vi "main.vi"() -> ()   [LabVIEW 2016]
uses:
  SALEvents/SAL_Events.lvclass
  SALListener/SAL_Listener.lvclass
  SALListener/SAL_Listener.lvclass/SAL_Listener.ctl
  SALEvents/SAL_Events.lvclass/SAL_Events.ctl
  SALLV_dome/DataTypes/command_start.ctl
  SALLV_dome/DataTypes/command_enable.ctl
  SALLV_dome/DataTypes/command_disable.ctl
  SALLV_dome/DataTypes/command_exitControl.ctl
  SALLV_dome/DataTypes/command_standby.ctl
  SALLV_dome/DataTypes/command_SetLouvers.ctl
  SALLV_dome/DataTypes/command_Move.ctl
  SALLV_dome/DataTypes/command_Crawl.ctl
  SALLV_dome/SALLV_dome.lvlib
panel:
  out "position_cmd":sgl
  out "position_actual":sgl
  out "position_error":sgl
  in  "Elevation":dbl
  in  "Azimuth":dbl
  in  "Crawl":bool
  in  "Move":bool
  in  "SetLouvers":bool
  in  "Array":i32[][](array[numeric])
  out "StateValue":string
  out "SummaryState":string
  in  "standby":bool
  in  "exitControl":bool
  in  "disable":bool
  in  "enable":bool
  in  "start":bool
  # "Main Controls"
  # "Louvers Command"
  # "States"
  # "Move Command"
  # "ADB Status"
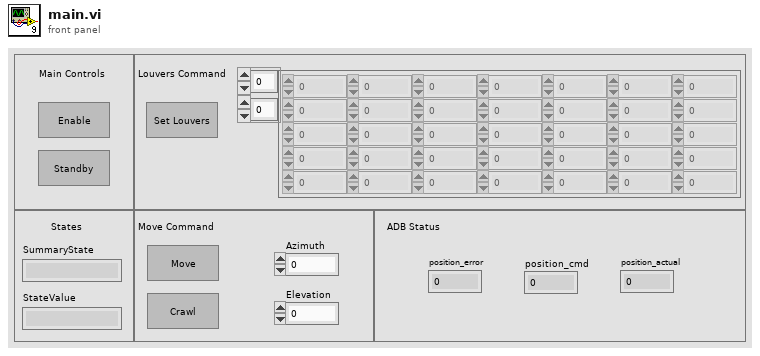
[diagram p1: front panel]
types:
  T1 = typedef "commandsEvents.ctl" = cluster{"start":refnum<user-event>, "disable":refnum<user-event>, "enable":refnum<user-event>, "exitControl":refnum<user-event>, "standby":refnum<user-event>, "stop":refnum<user-event>, "move":refnum<user-event>, "crawl":refnum<user-event>, "setLouvers":refnum<user-event>, "Park":refnum<user-event>, "StopShutter":refnum<user-event>, "OpenShutter":refnum<user-event>, "CloseShutter":refnum<user-event>}
  T2 = typedef "eventsEvents.ctl" = cluster{"AppliedSettingsMatchStart":refnum<user-event>, "ErrorCode":refnum<user-event>, "SettingVersions":refnum<user-event>, "StateChanged":refnum<user-event>, "SummaryState":refnum<user-event>}
  T3 = typedef "telemetryEvents.ctl" = cluster{"ADBstatus":refnum<user-event>}
  T4 = typedef "SALLV_dome.lvlib/command_start.ctl" = cluster{"configuration":string}
  T5 = typedef "SALLV_dome.lvlib/command_enable.ctl" = cluster{"state":bool}
  T6 = typedef "SALLV_dome.lvlib/command_disable.ctl" = cluster{"state":bool}
  T7 = typedef "SALLV_dome.lvlib/command_exitControl.ctl" = cluster{"state":bool}
  T8 = typedef "SALLV_dome.lvlib/command_standby.ctl" = cluster{"state":bool}
  T9 = typedef "SALLV_dome.lvlib/command_SetLouvers.ctl" = cluster{"position[34]":i32[]}
  T10 = typedef "SALLV_dome.lvlib/command_Move.ctl" = cluster{"azimuth":dbl, "elevation":dbl}
  T11 = typedef "SALLV_dome.lvlib/command_Crawl.ctl" = cluster{"azPosition":dbl, "elPosition":dbl, "demandTime":i32}
  T12 = enum16{"", "DisabledState", "EnabledState", "FaultState", "OfflineState", "StandbyState"}
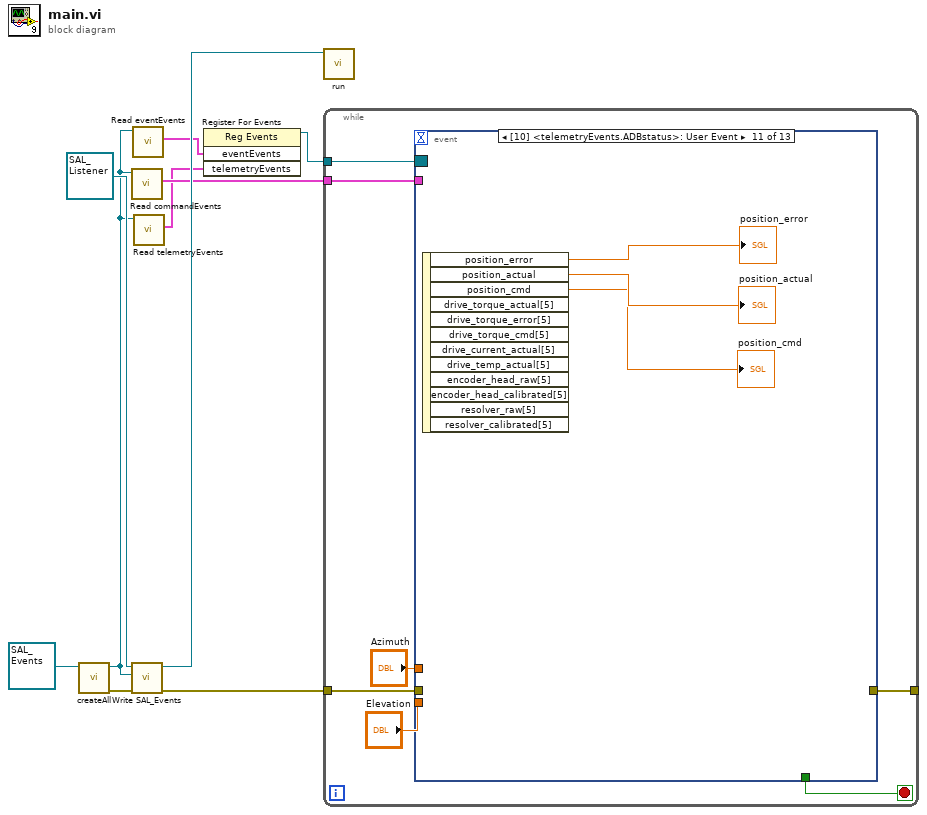
[diagram p0: block diagram]
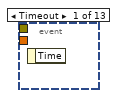
[diagram p2: hidden frame]
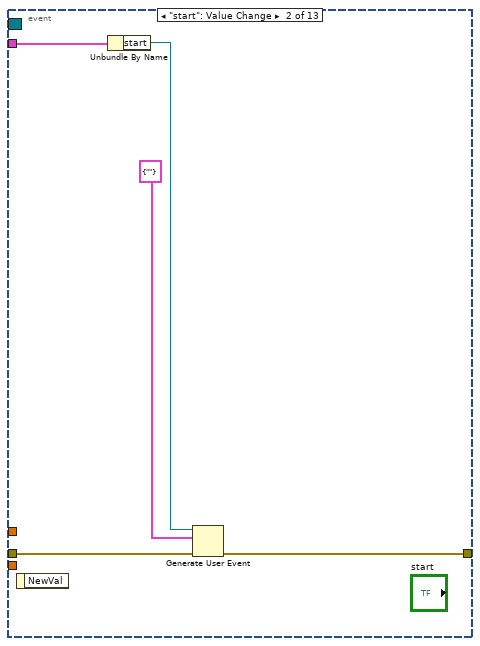
[diagram p3: hidden frame]
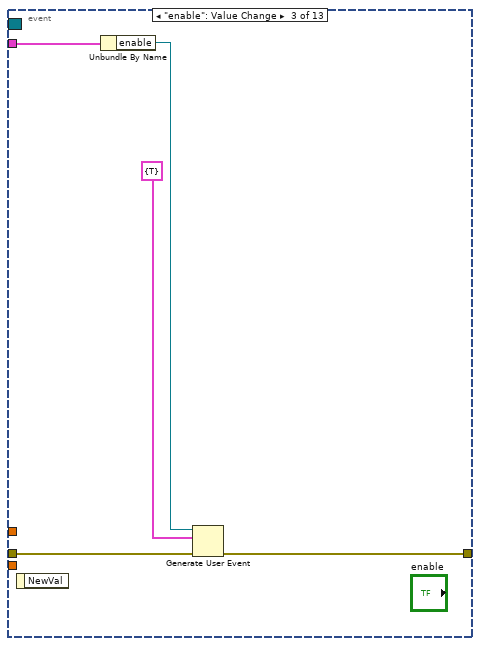
[diagram p4: hidden frame]
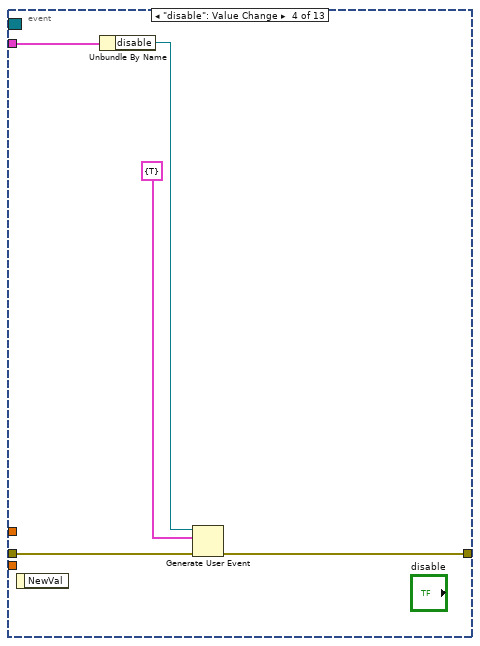
[diagram p5: hidden frame]
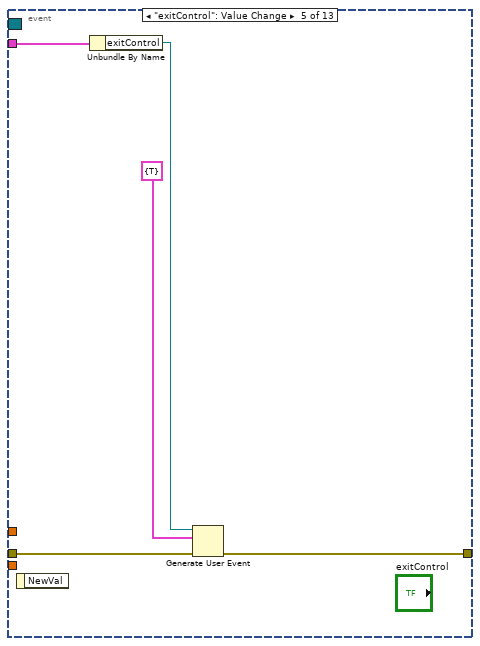
[diagram p6: hidden frame]
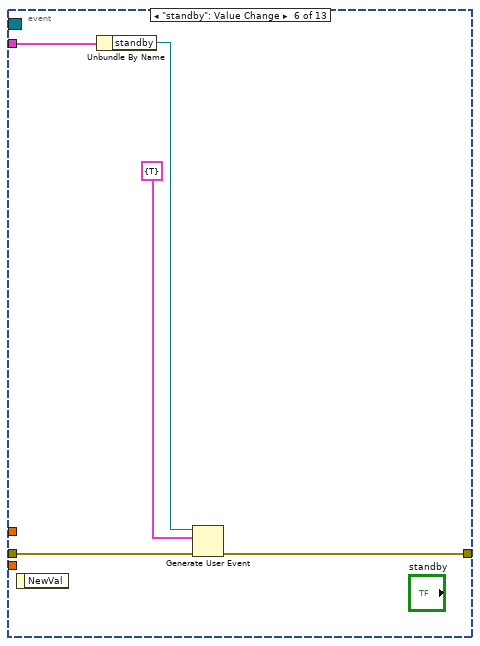
[diagram p7: hidden frame]
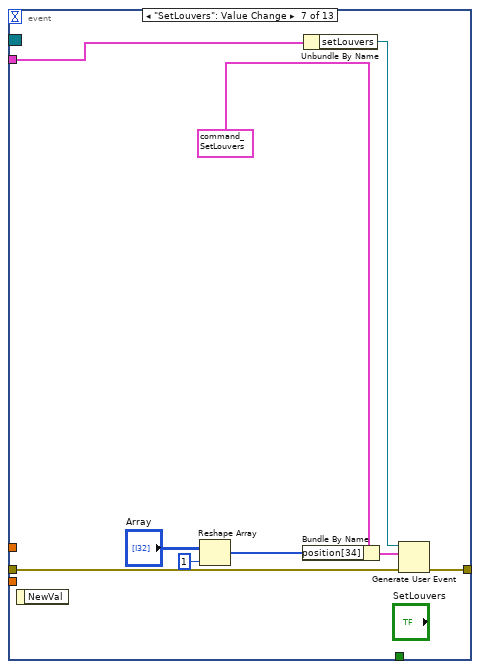
[diagram p8: hidden frame]
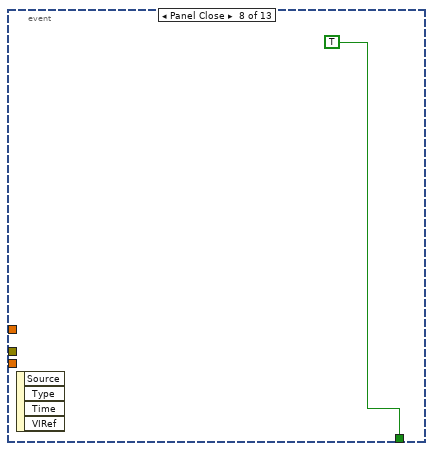
[diagram p9: hidden frame]
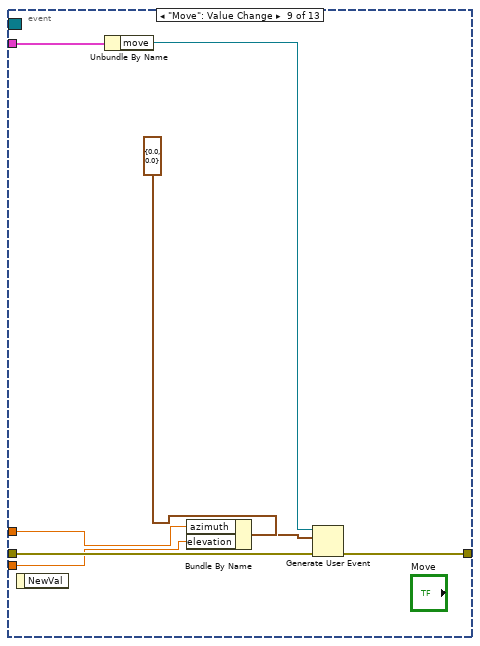
[diagram p10: hidden frame]
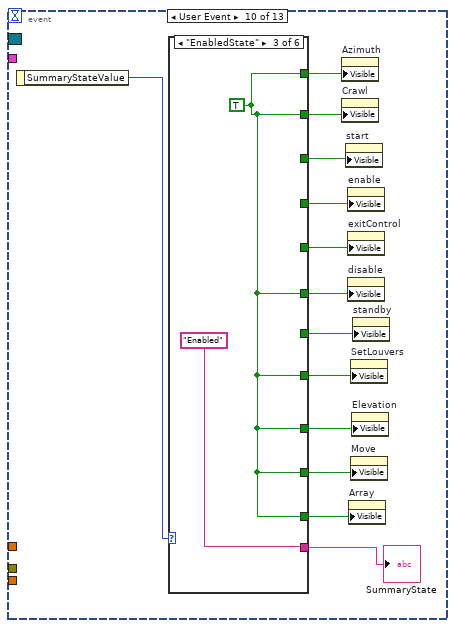
[diagram p11: hidden frame]
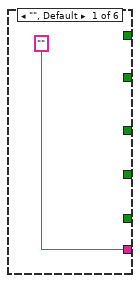
[diagram p12: hidden frame]
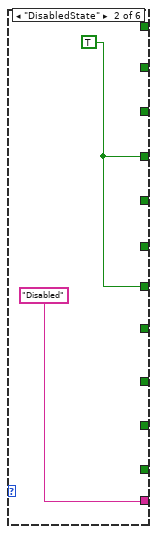
[diagram p13: hidden frame]
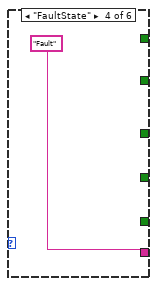
[diagram p14: hidden frame]
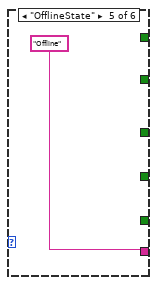
[diagram p15: hidden frame]
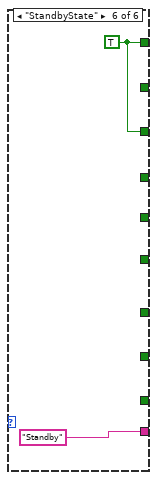
[diagram p16: hidden frame]
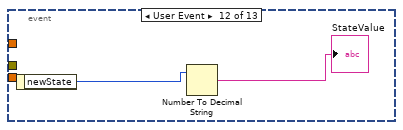
[diagram p17: hidden frame]
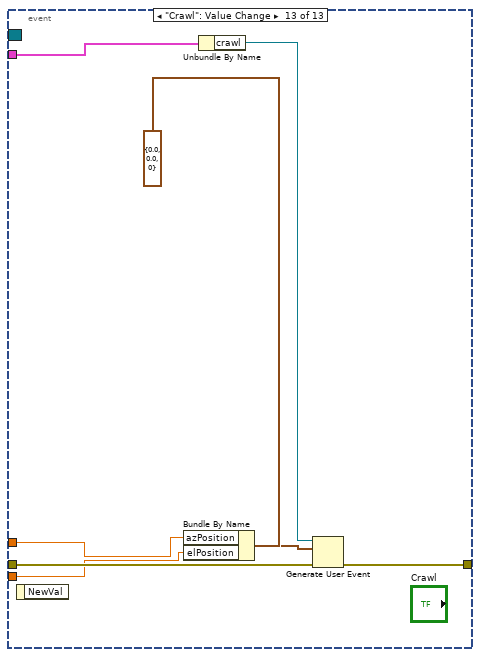
[diagram p18: hidden frame]
diagram:
  n1 = call "createAll.vi"("SAL_Events in"=refnum<class "SAL_Events.lvclass"> refnum ("SAL_Events.lvclass")) -> ("error out"=w7:errorcluster, "SAL_Events out"=w2:refnum<class "SAL_Events.lvclass">)  [unwired: 9 in]
  n2 = call "Read commandEvents.vi"("SAL_Events in"=w2) -> ("commandEvents"=w5:T1)  [unwired: 8 in, 2 out]
  n3 = call "Write SAL_Events.vi"("error in (no error)"=w7, "SAL_Events.lvclass"=w2, "SAL_Listener in"=refnum<class "SAL_Listener.lvclass"> refnum ("SAL_Listener.lvclass")) -> ("error out"=w6:errorcluster, "SAL_Listener out"=w8:refnum<class "SAL_Listener.lvclass">)  [unwired: 7 in]
  n4 = call "Read eventEvents.vi"("SAL_Events in"=w2) -> ("eventEvents"=w4:T2)  [unwired: 8 in, 2 out]
  n5 = call "Read telemetryEvents.vi"("SAL_Events in"=w2) -> ("telemetryEvents"=w1:T3)  [unwired: 8 in, 2 out]
  n6 = register-events(w4, w1) -> (reference out=w3:refnum<event-registration>)  [unwired: 2 in, 1 out]
  n7 = call "run.vi"("SAL_Listener in"=w8) -> ()  [unwired: 9 in, 2 out]
  n8 = while {
    tunnel: w6 -> [w16]
    tunnel: w5 -> [w17]
    tunnel: [w15] -> _
    tunnel: w3 -> [w12]
    stop <- w11 stop-if-true
    n9 = event shown="[10] <telemetryEvents.ADBstatus>: User Event" {
      selector: w12 -> [_ _ _ _ _ _ _ _ _ _ _ _ _]
      dyn-events: _ -> [_ _ _ _ _ _ _ _ _ _ _ _ _]
      timeout: _ -> [_ _ _ _ _ _ _ _ _ _ _ _ _]
      tunnel: w17 -> [_ w22 w27 w32 w37 w42 w51 _ w60 _ _ _ w95]
      tunnel: w16 -> [_ w19 w26 w29 w34 w39 w45 _ w58 _ _ _ w93]
      tunnel: [_ w18 w23 w28 w33 w38 w44 _ w57 _ _ _ w92] -> w15
      tunnel: "Azimuth" -> [_ _ _ _ _ _ _ _ w54 _ _ _ w89]
      tunnel: "Elevation" -> [_ _ _ _ _ _ _ _ w55 _ _ _ w88]
      tunnel: [_ _ _ _ _ _ _ TRUE _ _ _ _ _] -> w11
      event Timeout {
        n10 = event-data() -> ()  [unwired: 1 in, 1 out]
      }
      event "start": Value Change {
        n11 = event-data() -> ()  [unwired: 1 in, 1 out]
        n12 = Unbundle By Name(w22) -> ("start"=w21:refnum<user-event>)
        n13 = Generate User Event(user event=w21, event data cluster=T4 {"configuration"=""} ("event data"), error in=w19) -> (error out=w18:errorcluster)  [unwired: 1 in, 1 out]
      }
      event "enable": Value Change {
        n14 = event-data() -> ()  [unwired: 1 in, 1 out]
        n15 = Unbundle By Name(w27) -> ("enable"=w25:refnum<user-event>)
        n16 = Generate User Event(user event=w25, event data cluster=T5 {"state"=TRUE} ("event data"), error in=w26) -> (error out=w23:errorcluster)  [unwired: 1 in, 1 out]
      }
      event "disable": Value Change {
        n17 = event-data() -> ()  [unwired: 1 in, 1 out]
        n18 = Unbundle By Name(w32) -> ("disable"=w31:refnum<user-event>)
        n19 = Generate User Event(user event=w31, event data cluster=T6 {"state"=TRUE} ("event data"), error in=w29) -> (error out=w28:errorcluster)  [unwired: 1 in, 1 out]
      }
      event "exitControl": Value Change {
        n20 = event-data() -> ()  [unwired: 1 in, 1 out]
        n21 = Unbundle By Name(w37) -> ("exitControl"=w36:refnum<user-event>)
        n22 = Generate User Event(user event=w36, event data cluster=T7 {"state"=TRUE} ("event data"), error in=w34) -> (error out=w33:errorcluster)  [unwired: 1 in, 1 out]
      }
      event "standby": Value Change {
        n23 = event-data() -> ()  [unwired: 1 in, 1 out]
        n24 = Unbundle By Name(w42) -> ("standby"=w41:refnum<user-event>)
        n25 = Generate User Event(user event=w41, event data cluster=T8 {"state"=TRUE} ("event data"), error in=w39) -> (error out=w38:errorcluster)  [unwired: 1 in, 1 out]
      }
      event "SetLouvers": Value Change {
        n26 = event-data() -> ()  [unwired: 1 in, 1 out]
        n27 = Reshape Array("Array", 1 ("dimension size")) -> (w47:i32[])
        n28 = Bundle By Name(cluster=T9 {"position[34]"=[0, 0, 0, 0, 0, 0, 0, 0, 0, 0, 0, 0, 0, 0, 0, 0, 0, 0, 0, 0, 0, 0, 0, 0, 0, 0, 0, 0, 0, 0, 0, 0, 0, 0]} ("event data"), "position[34]"=w47) -> (w46:T9)
        n29 = Unbundle By Name(w51) -> ("setLouvers"=w50:refnum<user-event>)
        n30 = Generate User Event(user event=w50, event data cluster=w46, error in=w45) -> (error out=w44:errorcluster)  [unwired: 1 in, 1 out]
      }
      event Panel Close {
        n31 = event-data() -> ()  [unwired: 1 in, 4 out]
      }
      event "Move": Value Change {
        n32 = event-data() -> ()  [unwired: 1 in, 1 out]
        n33 = Unbundle By Name(w60) -> ("move"=w59:refnum<user-event>)
        n34 = Bundle By Name(cluster=T10 {"azimuth"=0.0, "elevation"=0.0} ("event data"), "azimuth"=w54, "elevation"=w55) -> (w53:T10)
        n35 = Generate User Event(user event=w59, event data cluster=w53, error in=w58) -> (error out=w57:errorcluster)  [unwired: 1 in, 1 out]
      }
      event User Event {
        n36 = event-data() -> ("SummaryStateValue"=w73:T12)  [unwired: 1 in]
        n37 = case shown="\"EnabledState\"" w73 {
          tunnel: ["" ("SummaryState") "Disabled" ("SummaryState") "Enabled" ("SummaryState") "Fault" ("SummaryState") "Offline" ("SummaryState") "Standby" ("SummaryState")] -> w72
          tunnel: [_ _ _ _ _ w81] -> w71
          tunnel: [_ _ _ _ _ w81] -> w70
          tunnel: [_ w75 _ _ _ _] -> w69
          tunnel: [_ w75 _ _ _ _] -> w68
          tunnel: [_ _ w77 _ _ _] -> w67
          tunnel: [_ _ w77 _ _ _] -> w66
          tunnel: [_ _ w77 _ _ _] -> w65
          tunnel: [_ _ w77 _ _ _] -> w64
          tunnel: [_ _ w77 _ _ _] -> w63
          tunnel: [_ _ w77 _ _ _] -> w62
          tunnel: [_ _ w77 _ _ _] -> w61
          frame "", Default {
          }
          frame "DisabledState" {
            w75 = TRUE ("Visible")
          }
          frame "EnabledState" {
            w77 = TRUE ("Visible")
          }
          frame "FaultState" {
          }
          frame "OfflineState" {
          }
          frame "StandbyState" {
            w81 = TRUE ("Visible")
          }
        }
        "SummaryState" <- w72
        n38 = property on="Azimuth" class="DigNum (strict)"("Visible"=w67) -> ()  [unwired: 2 in, 2 out]
        n39 = property on="Crawl" class="Bool"("Visible"=w66) -> ()  [unwired: 2 in, 2 out]
        n40 = property on="start" class="Bool"("Visible"=w71) -> ()  [unwired: 2 in, 2 out]
        n41 = property on="enable" class="Bool"("Visible"=w69) -> ()  [unwired: 2 in, 2 out]
        n42 = property on="exitControl" class="Bool"("Visible"=w70) -> ()  [unwired: 2 in, 2 out]
        n43 = property on="disable" class="Bool"("Visible"=w62) -> ()  [unwired: 2 in, 2 out]
        n44 = property on="Array" class="Arr (strict)"("Visible"=w61) -> ()  [unwired: 2 in, 2 out]
        n45 = property on="SetLouvers" class="Bool"("Visible"=w63) -> ()  [unwired: 2 in, 2 out]
        n46 = property on="Move" class="Bool"("Visible"=w64) -> ()  [unwired: 2 in, 2 out]
        n47 = property on="Elevation" class="DigNum (strict)"("Visible"=w65) -> ()  [unwired: 2 in, 2 out]
        n48 = property on="standby" class="Bool"("Visible"=w68) -> ()  [unwired: 2 in, 2 out]
      }
      event User Event {
        n49 = event-data() -> ("position_error"=→"position_error":sgl, "position_actual"=→"position_actual":sgl, "position_cmd"=→"position_cmd":sgl)  [unwired: 1 in, 9 out]
      }
      event User Event {
        n50 = event-data() -> ("newState"=w87:i32)  [unwired: 1 in]
        n51 = Number To Decimal String(number=w87) -> (decimal integer string=→"StateValue":string)  [unwired: 1 in]
      }
      event "Crawl": Value Change {
        n52 = event-data() -> ()  [unwired: 1 in, 1 out]
        n53 = Bundle By Name(cluster=T11 {"azPosition"=0.0, "elPosition"=0.0, "demandTime"=0} ("event data"), "azPosition"=w89, "elPosition"=w88) -> (w90:T11)
        n54 = Unbundle By Name(w95) -> ("crawl"=w94:refnum<user-event>)
        n55 = Generate User Event(user event=w94, event data cluster=w90, error in=w93) -> (error out=w92:errorcluster)  [unwired: 1 in, 1 out]
      }
    }
  }
